vi "Write object refs.vi"(8 "error in (no error)":errorcluster, 10 "references":T1, 11 "Table Manager in":refnum<class "Table Manager.lvclass">) -> (0 "error out":errorcluster, 3 "Table Manager out":refnum<class "Table Manager.lvclass">)   [LabVIEW 2013, in "Table Manager.lvlib" / "Table Manager.lvclass"]
uses:
  Table Manager.lvclass
  object ref.ctl
  Configuration Editor/Classes/Engine Parent/Engine Parent Editor Node.lvclass
  Configuration Editor/Classes/Module editor node/module editor node.lvclass
  Table Manager.lvclass/Table Manager.ctl
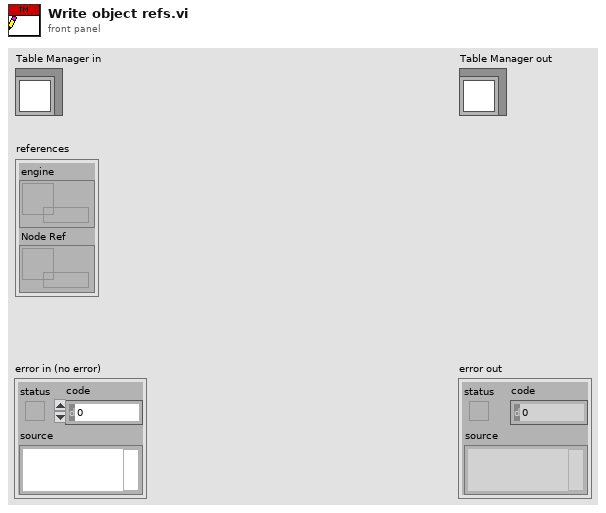
[diagram p1: front panel]
types:
  T1 = typedef "Table Manager.lvlib/Table Manager.lvclass/object ref.ctl" = cluster{"engine":refnum<data-value>, "Node Ref":refnum<data-value>}
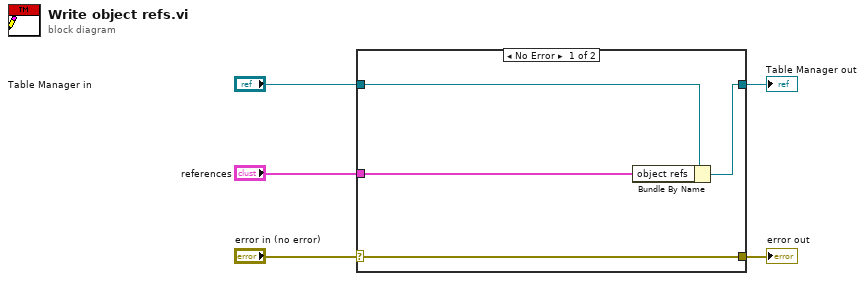
[diagram p0: block diagram]
diagram:
  n1 = case shown="No Error" "error in (no error)" {
    selector: "error in (no error)" -> [w9 w10]
    tunnel: [w9 w10] -> w4
    tunnel: [w7 w11] -> w2
    tunnel: "Table Manager in" -> [w8 w11]
    tunnel: "references" -> [w6 _]
    frame No Error {
      n2 = Bundle By Name(cluster=w8, "object refs"=w6) -> (w7:refnum<class "Table Manager.lvclass">)
    }
    frame Error {
    }
  }
  "error out" <- w4
  "Table Manager out" <- w2
